vi "CRYMicrophone Calibration by One.vi"() -> ()   [LabVIEW 2013]
uses:
  CRYSystem/Typedef Control/CRYCalibration All Cluster.ctl
  CRYSystem/Typedef Control/CRYCalibration 2DCluster.ctl
  CRYSystem/Typedef Control/CRYCalibration Cluster.ctl
  CRYSystem/Typedef Control/CRYData Cluster.ctl
  CRYSystem/Calibration/SubVI/CRYCal Global.vi
  CRYSystem/Misc/SubVI/CRYMisc vis settings global.vi
panel:
  in  "Hardware In":string
  in  "Calibration":T1 {"Calibration 2D"."Sens Curve"."Z data" items=["dB", "Lin"]; "Calibration 2D"."Sens Curve"."X data" items=["dB", "Lin"]; "Calibration 2D"."Sens Curve"."Y data" items=["dB", "Lin"]; "Calibration 2D"."Sens Curve"."Z dB ref" format="%.1f"; "Calibration 2D"."Sens Curve"."Z axis" items=["Log", "Lin"]; "Calibration 2D"."Sens Curve"."X dB ref" format="%.1f"; "Calibration 2D"."Sens Curve"."X axis" items=["Log", "Lin"]; "Calibration 2D"."Sens Curve"."Y axis" items=["Log", "Lin"]; "Calibration 2D"."Sens Curve"."Y dB ref" format="%.1f"; "Calibration 2D"."Sens Curve"."Curve"."z" format="%.2f"; "Calibration 2D"."Sens Curve"."Curve"."y" format="%.2f"; "Calibration 2D"."Sens Curve"."Curve"."x" format="%.2f"; "Calibration 2D"."EQ Curve"."Z data" items=["dB", "Lin"]; "Calibration 2D"."EQ Curve"."X data" items=["dB", "Lin"]; "Calibration 2D"."EQ Curve"."Y data" items=["dB", "Lin"]; "Calibration 2D"."EQ Curve"."Z dB ref" format="%.1f"; "Calibration 2D"."EQ Curve"."Z axis" items=["Log", "Lin"]; "Calibration 2D"."EQ Curve"."X dB ref" format="%.1f"; "Calibration 2D"."EQ Curve"."X axis" items=["Log", "Lin"]; "Calibration 2D"."EQ Curve"."Y axis" items=["Log", "Lin"]; "Calibration 2D"."EQ Curve"."Y dB ref" format="%.1f"; "Calibration 2D"."EQ Curve"."Curve"."z" format="%.2f"; "Calibration 2D"."EQ Curve"."Curve"."y" format="%.2f"; "Calibration 2D"."EQ Curve"."Curve"."x" format="%.2f"; "Calibration 2D"."Corr Curve"."Z data" items=["dB", "Lin"]; "Calibration 2D"."Corr Curve"."X data" items=["dB", "Lin"]; "Calibration 2D"."Corr Curve"."Y data" items=["dB", "Lin"]; "Calibration 2D"."Corr Curve"."Z dB ref" format="%.1f"; "Calibration 2D"."Corr Curve"."Z axis" items=["Log", "Lin"]; "Calibration 2D"."Corr Curve"."X dB ref" format="%.1f"; "Calibration 2D"."Corr Curve"."X axis" items=["Log", "Lin"]; "Calibration 2D"."Corr Curve"."Y axis" items=["Log", "Lin"]; "Calibration 2D"."Corr Curve"."Y dB ref" format="%.1f"; "Calibration 2D"."Corr Curve"."Curve"."z" format="%.2f"; "Calibration 2D"."Corr Curve"."Curve"."y" format="%.2f"; "Calibration 2D"."Corr Curve"."Curve"."x" format="%.2f"; "Calibration 2D"."Calibration"."EQ Step size" items=["R10", "R20", "R40", "R80", "User"]; "Calibration 2D"."Calibration"."Corr Step size" items=["R10", "R20", "R40", "R80", "User"]}
  in  "Proper VI No In":i32
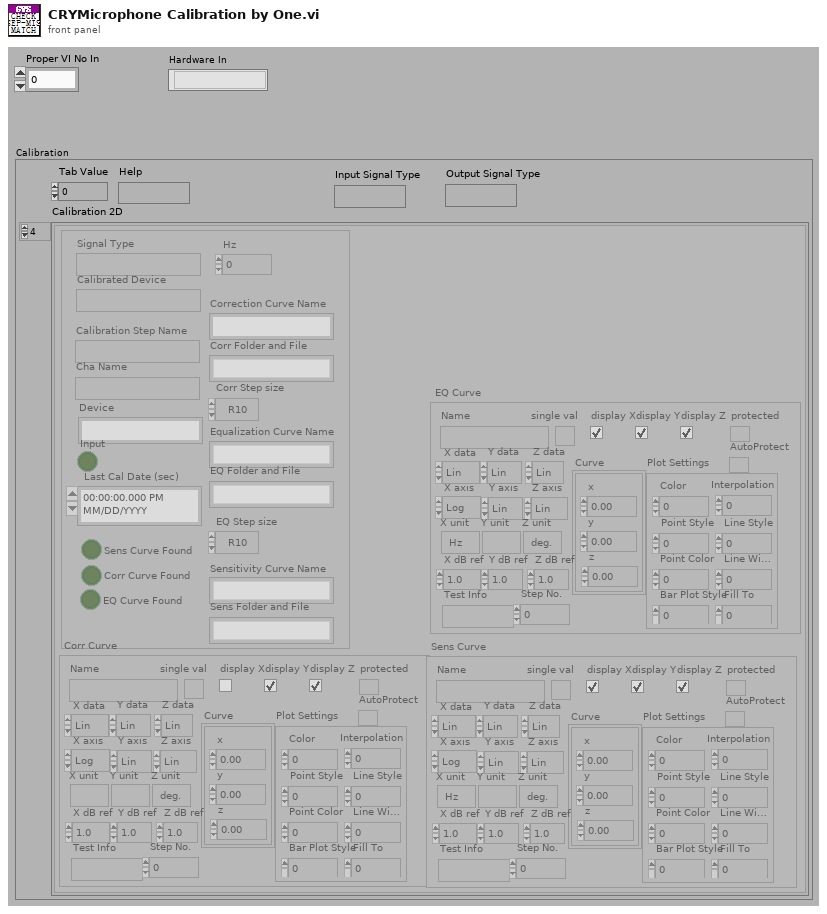
[diagram p1: front panel]
types:
  T1 = typedef "CRYCalibration All Cluster.ctl" = cluster{"Calibration 2D":T2[], "Help":string, "Tab Value":i32, "Input Signal Type":string, "Output Signal Type":string}
  T2 = typedef "CRYCalibration 2DCluster.ctl" = cluster{"Calibration":T3, "Corr Curve":T4, "EQ Curve":T4, "Sens Curve":T4}
  T3 = typedef "CRYCalibration Cluster.ctl" = cluster{"Calibration Step Name":string, "Device":string, "Correction Curve Name":string, "Equalization Curve Name":string, "Sensitivity Curve Name":string, "Corr Folder and File":string, "EQ Folder and File":string, "Sens Folder and File":string, "Corr Step size":u16, "EQ Step size":u16, "Input":bool, "Last Cal Date (sec)":timestamp, "Cha Name":string, "Corr Curve Found":bool, "EQ Curve Found":bool, "Sens Curve Found":bool, "Signal Type":string, "Calibrated Device":string, "Hz":u32}
  T4 = typedef "CRYData Cluster.ctl" = cluster{"Name":string, "Curve":cluster{"x":dbl, "y":dbl, "z":dbl}[], "X data":u16, "Y data":u16, "Z data":u16, "X axis":u16, "Y axis":u16, "Z axis":u16, "X unit":string, "Y unit":string, "Z unit":string, "X dB ref":dbl, "Y dB ref":dbl, "Z dB ref":dbl, "single val":bool, "protected":bool, "display X":bool, "display Y":bool, "display Z":bool, "Test Info":string, "Step No.":i32, "Plot Settings":cluster{"Color":u32, "Interpolation":u8, "Point Style":u8, "Line Style":u8, "Point Color":u32, "Line Width":u8, "Bar Plot Style":u8, "Fill To":i16}, "AutoProtect":bool}
  T5 = cluster{"gen'r mode":i32, "frequency":u32, "output level":dbl, "wave path":string, "wav play mode":i32, "duration":dbl, "n times":i32, "channel":i32, "wav level":dbl, "EQ":bool, "f knob log":bool, "f knob low":dbl, "f knob high":dbl, "ol knob log":bool, "ol knob low":dbl, "ol knob high":dbl, "Lin Display Prefs":string, "dB Display Prefs":string, "Duration noise":dbl, "Min freq noise":dbl, "Max freq noise":dbl, "Signal Type":string, "Play Sine Wave":i32}
  T6 = typedef "CRYMultimeter.ctl" = cluster{"Ave/Max/Min":i32, "Level":i32, "Channel":i32, "Signal Type":string, "Weighting":string, "Applay Correction":bool, "lin/exp avg":u16, "rec time (sec)":dbl, "Average Time (Sec)":dbl, "Lin Display Prefs":string, "dB Display Prefs":string, "Time Weighting":u16, "Display":u16}
  T7 = typedef "CRYHardware Channel Info.ctl" = cluster{"ID":i32, "Name":string, "Digital":bool, "Input":bool, "Device Name":string, "Hardware Ch ID":u8, "Vmax (V)":dbl, "Latency (samples)":dbl, "Sampling Rate (Hz)":u32, "Bit Depth":u32, "Anti-aliasing Factor (%fs)":sgl, "DAQmx Channel":tag, "term config":i32, "Coupling":i32, "IEPE en":bool, "ASIOChannel Name":string, "Audio Driver":u16, "ASIOChannel Index":u8}
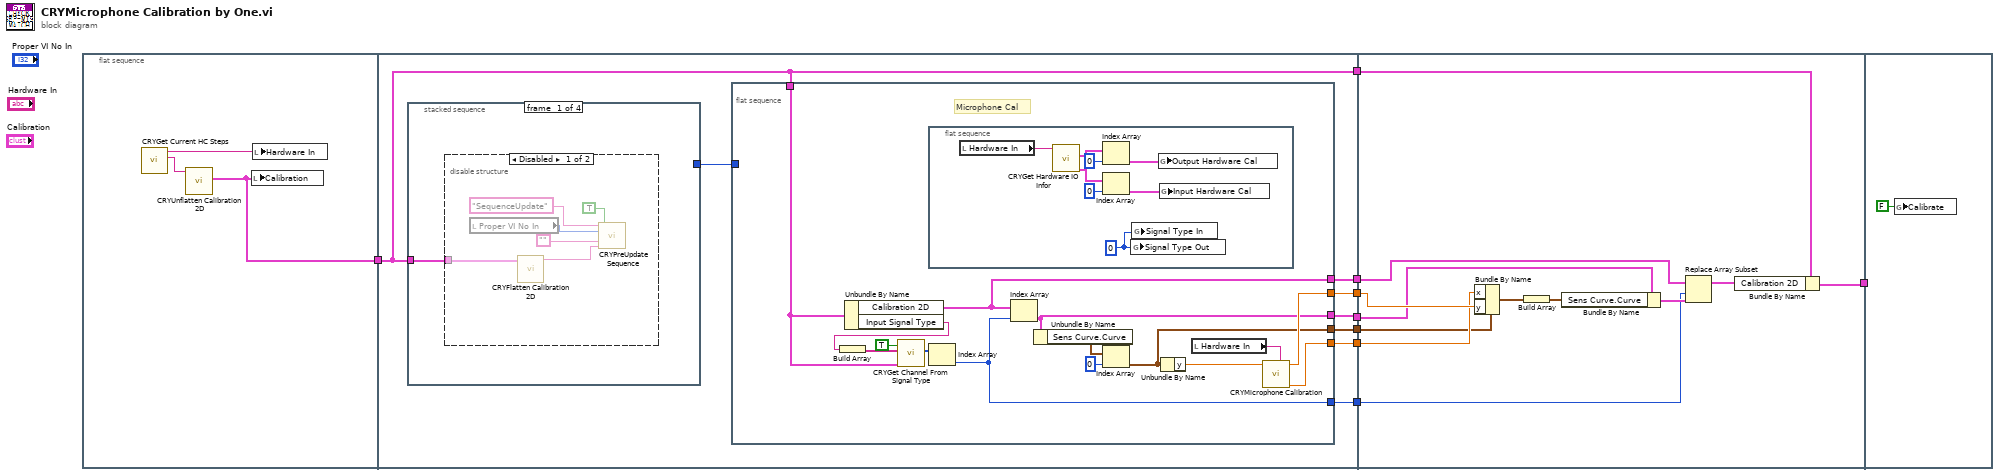
[diagram p0: block diagram]
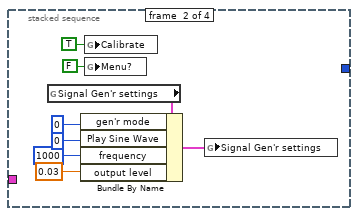
[diagram p3: hidden frame]
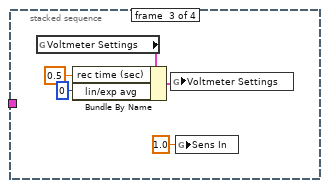
[diagram p4: hidden frame]
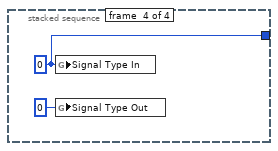
[diagram p5: hidden frame]
diagram:
  n1 = flat-sequence {
    tunnel: [w10] -> w1
    tunnel: [w20] -> w9
    tunnel: [w19] -> w8
    tunnel: [w18] -> w7
    tunnel: [w17] -> w6
    tunnel: [w16] -> w5
    tunnel: [w15] -> w4
    tunnel: [w13] -> w3
    tunnel: w1 -> [w13]
    tunnel: w9 -> [w74]
    tunnel: w8 -> [w72]
    tunnel: w7 -> [w69]
    tunnel: w6 -> [w71]
    tunnel: w5 -> [w70]
    tunnel: w4 -> [w68]
    tunnel: w3 -> [w67]
    tunnel: [w66] -> w2
    tunnel: w2 -> [_]
    frame #0 {
      n2 = call "CRYGet Current HC Steps.vi"() -> ("Calibration setup flattened Out"=w11:string, "Hardware setup flattened Out"=w12:string)  [unwired: 10 in]
      n3 = call "CRYUnflatten Calibration 2D.vi"("Flattened Calibration"=w11) -> ("Calibration Step Out"=w10:T1)  [unwired: 2 in, 8 out]
      n4 = local write "Calibration"(w10) -> ()
      n5 = local write "Hardware In"(w12) -> ()
    }
    frame #1 {
      n6 = stacked-sequence {
        tunnel: w13 -> [w44 _ _ _]
        tunnel: [_ _ _ w64] -> w14
        frame #0 {
          n7 = disable-structure shown="Disabled" {
            disable-tunnel: w44 -> [w45 _]
            frame Disabled {
              n8 = local read "Proper VI No In"() -> (w49:i32)
              n9 = call "CRYFlatten Calibration 2D.vi"("Calibration All Cluster"=w45) -> ("Calibration flattened"=w46:string)  [unwired: 10 in]
              n10 = call "CRYPreUpdate Sequence.vi"("EventName"="SequenceUpdate", "Proper VI No"=w49, "Project View Step Name Identifier Arg1"="", "Step flattened Arg2"=w46, "AllChangeFlg"=TRUE ("Name/Identifier")) -> ()  [unwired: 11 in]
            }
            frame Enabled {
            }
          }
        }
        frame #1 {
          n11 = global read "CRYMisc vis settings global.vi" "Signal Gen'r settings"() -> (w57:T5)
          n12 = Bundle By Name(cluster=w57, "gen'r mode"=0, "Play Sine Wave"=0, "frequency"=u32 1000, "output level"=0.03) -> (w52:T5)
          n13 = global write "CRYCal Global.vi" "Calibrate"(TRUE ("Calibrate")) -> ()
          n14 = global write "CRYMisc vis settings global.vi" "Menu?"(FALSE ("Menu?")) -> ()
          n15 = global write "CRYMisc vis settings global.vi" "Signal Gen'r settings"(w52) -> ()
        }
        frame #2 {
          n16 = global read "CRYMisc vis settings global.vi" "Voltmeter Settings"() -> (w62:T6)
          n17 = Bundle By Name(cluster=w62, "rec time (sec)"=0.5, "lin/exp avg"=u16 0) -> (w61:T6)
          n18 = global write "CRYMisc vis settings global.vi" "Voltmeter Settings"(w61) -> ()
          n19 = global write "CRYCal Global.vi" "Sens In"(1.0 ("Sens In")) -> ()
        }
        frame #3 {
          w64 = u16 0 ("Signal Type In")
          n20 = global write "CRYCal Global.vi" "Signal Type In"(w64) -> ()
          n21 = global write "CRYCal Global.vi" "Signal Type Out"(u16 0 ("Signal Type Out")) -> ()
        }
      }
      n22 = flat-sequence {
        tunnel: [w34] -> w20
        tunnel: [w33] -> w19
        tunnel: w13 -> [w27]
        tunnel: [w24] -> w18
        tunnel: [w23] -> w17
        tunnel: [w22] -> w16
        tunnel: [w21] -> w15
        tunnel: w14 -> [_]
        frame #0 {
          # "Microphone Cal"
          n23 = Unbundle By Name(w27) -> ("Calibration 2D"=w21:T2[], "Input Signal Type"=w26:string)
          n24 = Build Array(w26) -> (w28:string[])
          n25 = call "CRYGet Channel From Signal Type.vi"("Calibration"=w27, "Signal Type Name Array In"=w28, "In/Out?"=TRUE) -> ("equal Index Out"=w30:i32[])  [unwired: 7 in, 1 out]
          n26 = flat-sequence {
            frame #0 {
              w43 = u16 0 ("Signal Type In")
              n27 = local read "Hardware In"() -> (w38:string)
              n28 = call "CRYGet Hardware IO Infor.vi"("Hardware setup In"=w38) -> ("I_channel Info Out"=w40:T7[], "O_channel Info Out"=w39:T7[])  [unwired: 9 out]
              n29 = Index Array(array=w39, index=0) -> (element=w41:T7)
              n30 = Index Array(array=w40, index=0) -> (element=w42:T7)
              n31 = global write "CRYCal Global.vi" "Signal Type Out"(w43) -> ()
              n32 = global write "CRYCal Global.vi" "Signal Type In"(w43) -> ()
              n33 = global write "CRYCal Global.vi" "Output Hardware Cal"(w41) -> ()
              n34 = global write "CRYCal Global.vi" "Input Hardware Cal"(w42) -> ()
            }
          }
          n35 = Index Array(array=w30) -> (element=w22:i32)  [unwired: 1 in]
          n36 = Index Array(array=w21, index=w22) -> (element=w24:T2)
          n37 = Unbundle By Name(w24) -> ("Sens Curve.Curve"=w31:cluster{"x":dbl, "y":dbl, "z":dbl}[])
          n38 = Index Array(array=w31, index=0) -> (element=w23:cluster{"x":dbl, "y":dbl, "z":dbl})
          n39 = Unbundle By Name(w23) -> ("y"=w25:dbl)
          n40 = local read "Hardware In"() -> (w35:string)
          n41 = call "CRYMicrophone Calibration.vi"("Hardware in"=w35, "Old Total Sens"=w25) -> ("Ref. Freq out"=w33:dbl, "Total Sens"=w34:dbl)  [unwired: 3 in, 5 out]
        }
      }
    }
    frame #2 {
      n42 = Bundle By Name(cluster=w71, "x"=w72, "y"=w74) -> (w77:cluster{"x":dbl, "y":dbl, "z":dbl})
      n43 = Build Array(w77) -> (w76:cluster{"x":dbl, "y":dbl, "z":dbl}[])
      n44 = Bundle By Name(cluster=w69, "Sens Curve.Curve"=w76) -> (w75:T2)
      n45 = Replace Array Subset(array=w68, new element=w75, index=w70) -> (w73:T2[])
      n46 = Bundle By Name(cluster=w67, "Calibration 2D"=w73) -> (w66:T1)
    }
    frame #3 {
      n47 = global write "CRYCal Global.vi" "Calibrate"(FALSE ("Calibrate")) -> ()
    }
  }
